vi "WriteToSI.vi"(8 "SI camera info":T1, 11 "Refnum in":refnum<vi>) -> (0 "error out":errorcluster, 3 "Refnum out":refnum<vi>)   [LabVIEW 2015]
uses:
  Systems/SIcamera_Control/SIcamera_Globals.vi
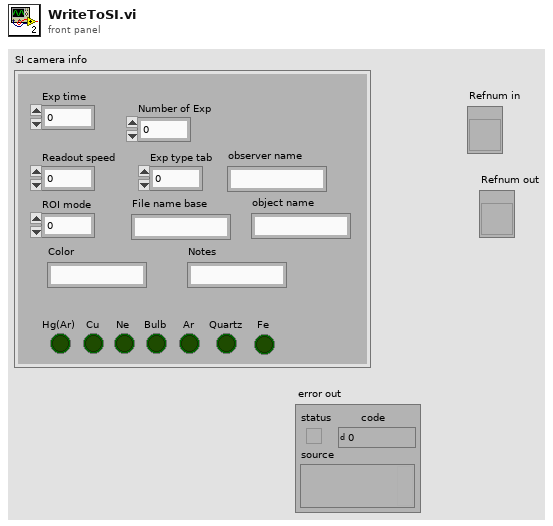
[diagram p1: front panel]
types:
  T1 = cluster{"Exp time":dbl, "Number of Exp":dbl, "Readout speed":dbl, "Exp type tab":dbl, "ROI mode":dbl, "File name base":string, "Color":string, "Notes":string, "observer name":string, "object name":string, "Hg(Ar)":bool, "Cu":bool, "Ne":bool, "Ar":bool, "Quartz":bool, "Fe":bool, "Bulb":bool}
  T2 = cluster{"ROI Mode":refnum<vi>, "RO Speed":refnum<vi>, "File name":refnum<vi>, "Exp time":refnum<vi>, "Start exp":refnum<vi>, "num exp":refnum<vi>, "cam color":refnum<vi>, "Exp tab":refnum<vi>, "notes":refnum<vi>, "observer name":refnum<vi>, "object name":refnum<vi>, "Ar":refnum<vi>, "Bulb":refnum<vi>, "Fe":refnum<vi>, "Hg(Ar)":refnum<vi>, "Cu":refnum<vi>, "Ne":refnum<vi>, "Quartz":refnum<vi>}
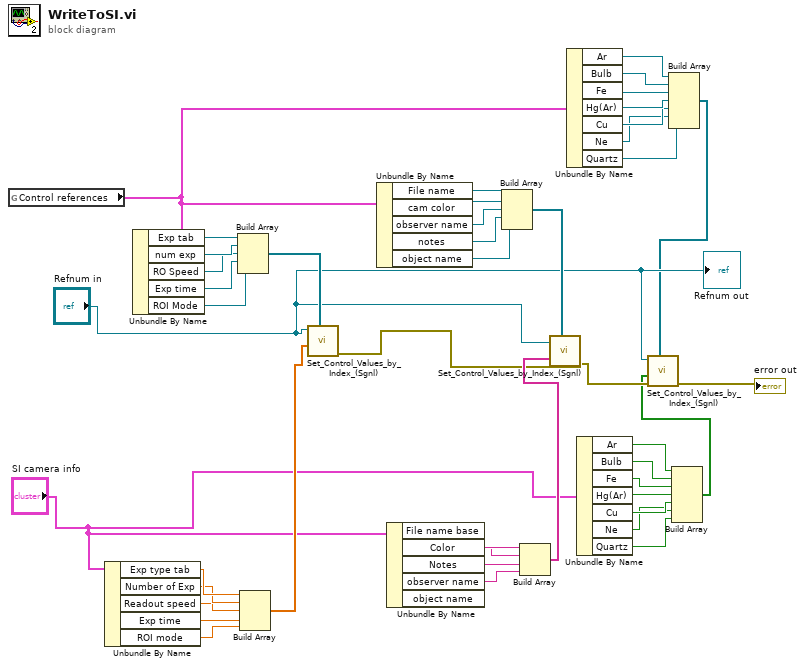
[diagram p0: block diagram]
diagram:
  n1 = global read "SIcamera_Globals.vi" "Control references"() -> (w18:T2)
  n2 = Unbundle By Name("SI camera info") -> ("Exp type tab"=w45:dbl, "Number of Exp"=w44:dbl, "Readout speed"=w43:dbl, "Exp time"=w42:dbl, "ROI mode"=w41:dbl)
  n3 = Unbundle By Name(w18) -> ("Exp tab"=w24:refnum<vi>, "num exp"=w33:refnum<vi>, "RO Speed"=w32:refnum<vi>, "Exp time"=w31:refnum<vi>, "ROI Mode"=w30:refnum<vi>)
  n4 = Build Array(w24, w33, w32, w31, w30) -> (w23:refnum<vi>[])
  n5 = Build Array(w45, w44, w43, w42, w41) -> (w36:dbl[])
  n6 = call "Set_Control_Values_by_Index_(Sgnl).vi"("Control References"=w23, "appended array"=w36, "VI Refnum"="Refnum in") -> ("error out"=w34:errorcluster)  [unwired: 8 in]
  n7 = Unbundle By Name(w18) -> ("File name"=w29:refnum<vi>, "cam color"=w28:refnum<vi>, "observer name"=w27:refnum<vi>, "notes"=w26:refnum<vi>, "object name"=w25:refnum<vi>)
  n8 = Unbundle By Name("SI camera info") -> ("File name base"=w40:string, "Color"=w39:string, "Notes"=w38:string, "observer name"=w37:string)  [unwired: 1 out]
  n9 = Build Array(w29, w28, w27, w26, w25) -> (w22:refnum<vi>[])
  n10 = Build Array(w40, w39, w38, w37) -> (w35:string[])
  n11 = call "Set_Control_Values_by_Index_(Sgnl).vi"("Control References"=w22, "error in (no error)"=w34, "appended array"=w35, "VI Refnum"="Refnum in") -> ("error out"=w21:errorcluster)  [unwired: 7 in]
  n12 = Unbundle By Name(w18) -> ("Ar"=w17:refnum<vi>, "Bulb"=w16:refnum<vi>, "Fe"=w15:refnum<vi>, "Hg(Ar)"=w14:refnum<vi>, "Cu"=w13:refnum<vi>, "Ne"=w12:refnum<vi>, "Quartz"=w11:refnum<vi>)
  n13 = Unbundle By Name("SI camera info") -> ("Ar"=w9:bool, "Bulb"=w8:bool, "Fe"=w7:bool, "Hg(Ar)"=w6:bool, "Cu"=w5:bool, "Ne"=w4:bool, "Quartz"=w3:bool)
  n14 = Build Array(w17, w16, w15, w14, w13, w12, w11) -> (w10:refnum<vi>[])
  n15 = Build Array(w9, w8, w7, w6, w5, w4, w3) -> (w2:bool[])
  n16 = call "Set_Control_Values_by_Index_(Sgnl).vi"("Control References"=w10, "error in (no error)"=w21, "appended array"=w2, "VI Refnum"="Refnum in") -> ("error out"=→"error out":errorcluster)  [unwired: 7 in]
  "Refnum out" <- "Refnum in"
